vi "ziTC2BW.vi"(1 "Eq BW (F)":bool, 2 "Order (1)":i32=1, 3 "TC (s)":dbl=1.0) -> (0 "BW (Hz)":dbl)   [LabVIEW 2018, in "Zurich Instruments LabOne.lvlib"]
doc: "Convert a timeconstant value and order value to an effective signal bandwidth.\nThe signal bandwidth is defined by 3dB points.\n\n<B>Order</B> range: 1 to 8\n<B>Eq BW</B> true: calculate equivalent-power BW; false: caluclate signal bandwidth"
uses:
  Zurich Instruments LabOne.lvlib
panel:
  out "Numeric":dbl
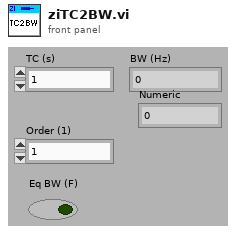
[diagram p1: front panel]
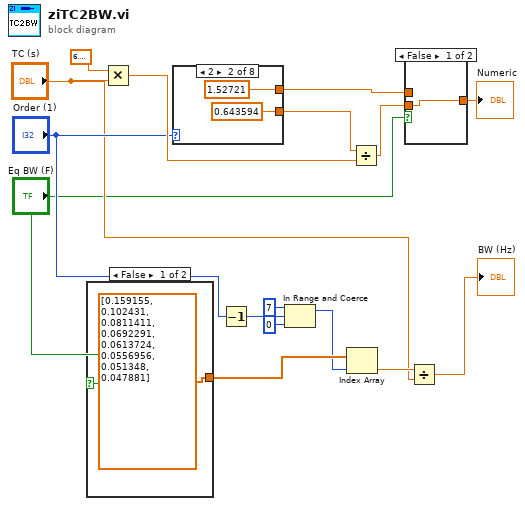
[diagram p0: block diagram]
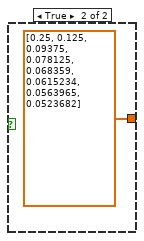
[diagram p2: hidden frame]
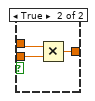
[diagram p3: hidden frame]
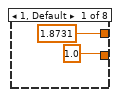
[diagram p4: hidden frame]
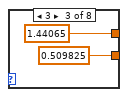
[diagram p5: hidden frame]
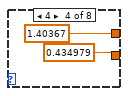
[diagram p6: hidden frame]
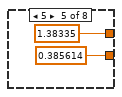
[diagram p7: hidden frame]
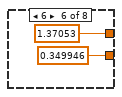
[diagram p8: hidden frame]
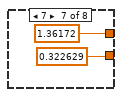
[diagram p9: hidden frame]
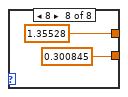
[diagram p10: hidden frame]
diagram:
  n1 = case shown="False" "Eq BW (F)" {
    tunnel: [dbl[] [0.159155, 0.102431, 0.0811411, 0.0692291, 0.0613724, 0.0556956, 0.051348, 0.047881] dbl[] [0.25, 0.125, 0.09375, 0.078125, 0.068359, 0.0615234, 0.0563965, 0.0523682]] -> w4
    frame False {
    }
    frame True {
    }
  }
  n2 = Multiply(x=6.283185307179586, y="TC (s)") -> (x*y=w14:dbl)
  n3 = case shown="2" "Order (1)" {
    tunnel: [1.0 ("y") 0.643594 ("y") 0.509825 ("y") 0.434979 ("y") 0.385614 ("y") 0.349946 ("y") 0.322629 ("y") 0.300845 ("y")] -> w15
    tunnel: [1.8731 ("y") 1.52721 ("y") 1.44065 ("y") 1.40367 ("y") 1.38335 ("y") 1.37053 ("y") 1.36172 ("y") 1.35528 ("y")] -> w13
    frame 1, Default {
    }
    frame 2 {
    }
    frame 3 {
    }
    frame 4 {
    }
    frame 5 {
    }
    frame 6 {
    }
    frame 7 {
    }
    frame 8 {
    }
  }
  n4 = Decrement(x="Order (1)") -> (x-1=w5:i32)
  n5 = In Range and Coerce(upper limit=7, x=w5, lower limit=0) -> (coerced(x)=w3:i32)  [unwired: 1 out]
  n6 = Index Array(array=w4, index=w3) -> (element=w10:dbl)
  n7 = Divide(x=w15, y=w14) -> (x/y=w16:dbl)
  n8 = case shown="False" "Eq BW (F)" {
    tunnel: w16 -> [w35 w38]
    tunnel: [w35 w37] -> w1
    tunnel: w13 -> [_ w36]
    frame False {
    }
    frame True {
      n9 = Multiply(x=w36, y=w38) -> (x*y=w37:dbl)
    }
  }
  "Numeric" <- w1
  n10 = Divide(x=w10, y="TC (s)") -> (x/y=→"BW (Hz)":dbl)
